vi "tacking_points.vi"(9 "NotifierReff":T1, 10 "Waypoint queue":refnum<queue>) -> (2 "size(s)":i32, 3 "New Sailing points":refnum<class "Waypoint.lvclass">[](array[class]), 5 "Waypoint Queue Out":refnum<queue>)   [LabVIEW 2013]
doc: "Creates tacking point or points nessisary to reach waypoint from current position. \n\n- (11/8/2014) Kaitlin Gallagher"
uses:
  Data/TypeDefs/Notifiers.ctl
  Data/TypeDefs/UTM Location.ctl
  Data/TypeDefs/Sail Set Suggestions.ctl
  Data/TypeDefs/Rudder Set Suggestions.ctl
  Data/TypeDefs/OverrideInformation.ctl
  Data/TypeDefs/OverrideMode.ctl
  Data/TypeDefs/MotorSetup.ctl
  Data/TypeDefs/DynamixelSetupInfo.ctl
  Data/TypeDefs/AirmarStatus.ctl
  Data/TypeDefs/HardwareOnline.ctl
  Data/TypeDefs/DynamixelCycleTracker.ctl
  Data/TypeDefs/RC Input Values.ctl
  Classes/Waypoint/Waypoint.lvclass
panel:
  in  "Coridor Width":dbl=100.0
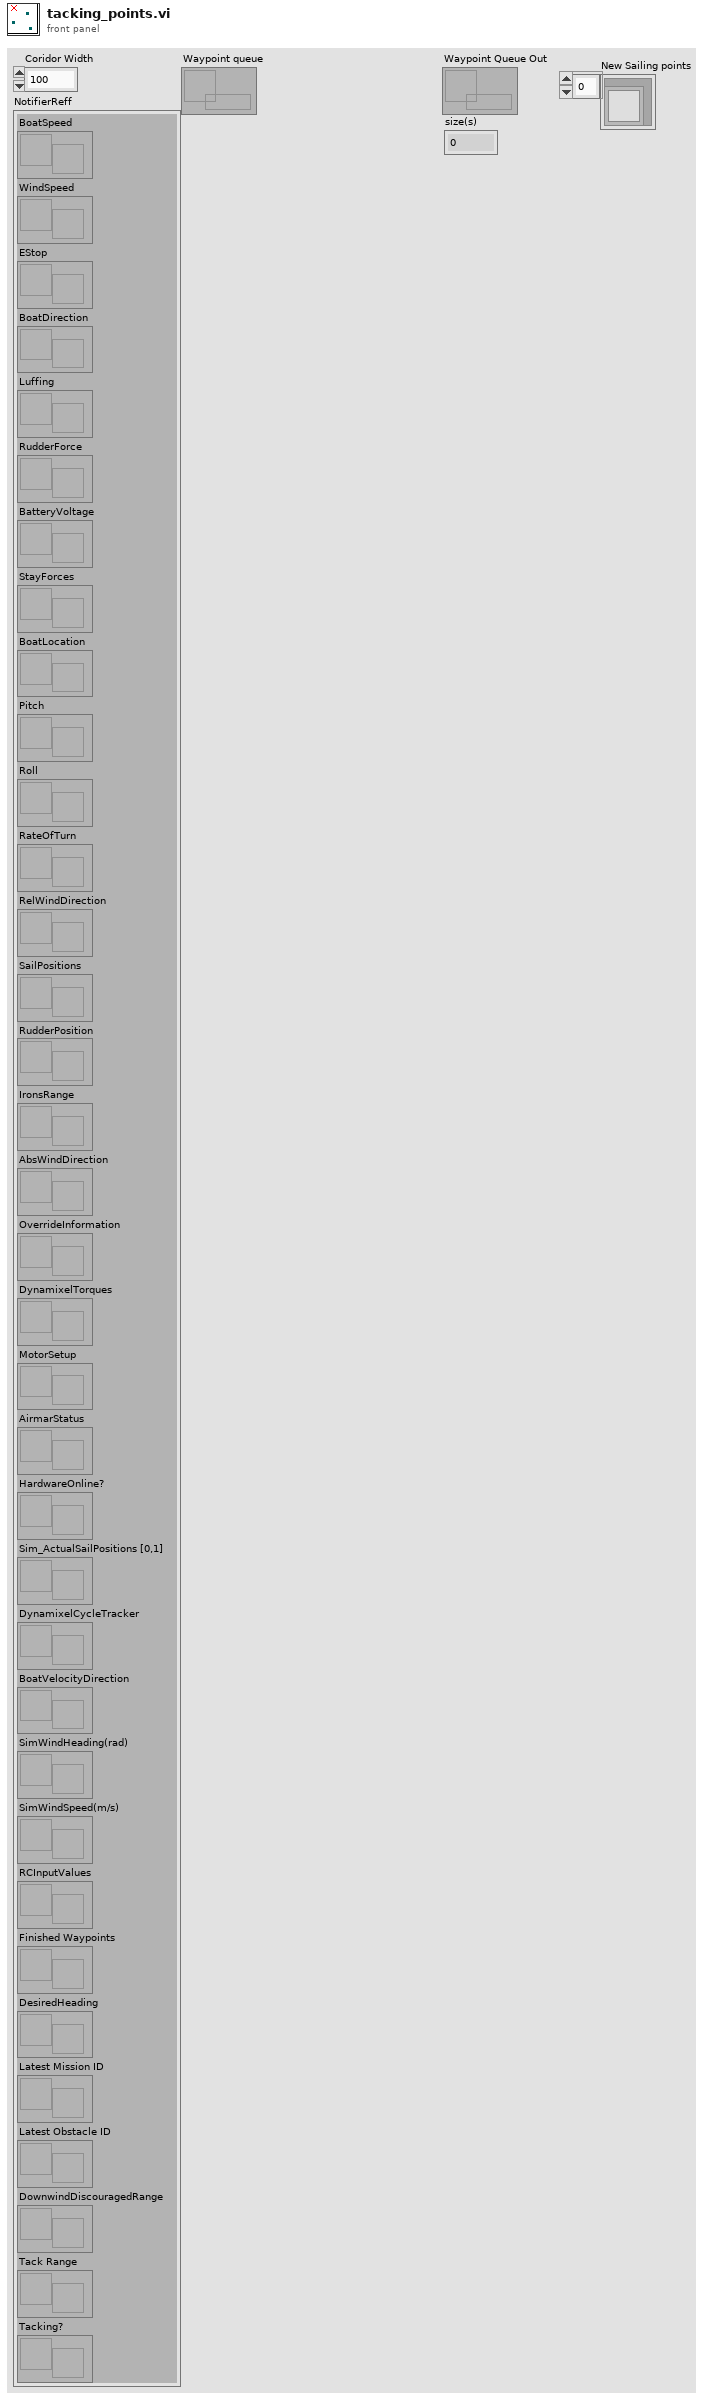
[diagram p1: front panel]
types:
  T1 = typedef "Notifiers.ctl" = cluster{"BoatSpeed":refnum<notifier>, "WindSpeed":refnum<notifier>, "EStop":refnum<notifier>, "BoatDirection":refnum<notifier>, "Luffing":refnum<notifier>, "RudderForce":refnum<notifier>, "BatteryVoltage":refnum<notifier>, "StayForces":refnum<notifier>, "BoatLocation":refnum<notifier>, "Pitch":refnum<notifier>, "Roll":refnum<notifier>, "RateOfTurn":refnum<notifier>, "RelWindDirection":refnum<notifier>, "SailPositions":refnum<notifier>, "RudderPosition":refnum<notifier>, "IronsRange":refnum<notifier>, "AbsWindDirection":refnum<notifier>, "OverrideInformation":refnum<notifier>, "DynamixelTorques":refnum<notifier>, "MotorSetup":refnum<notifier>, "AirmarStatus":refnum<notifier>, "HardwareOnline?":refnum<notifier>, "Sim_ActualSailPositions [0,1]":refnum<notifier>, "DynamixelCycleTracker":refnum<notifier>, "BoatVelocityDirection":refnum<notifier>, "SimWindHeading(rad)":refnum<notifier>, "SimWindSpeed(m/s)":refnum<notifier>, "RCInputValues":refnum<notifier>, "Finished Waypoints":refnum<notifier>, "DesiredHeading":refnum<notifier>, "Latest Mission ID":refnum<notifier>, "Latest Obstacle ID":refnum<notifier>, "DownwindDiscouragedRange":refnum<notifier>, "Tack Range":refnum<notifier>, "Tacking?":refnum<notifier>}
  T2 = typedef "UTM Location.ctl" = cluster{"UTM Zone":dbl, "Hemisphere":enum16{"North", "South"}, "East":dbl, "North":dbl}
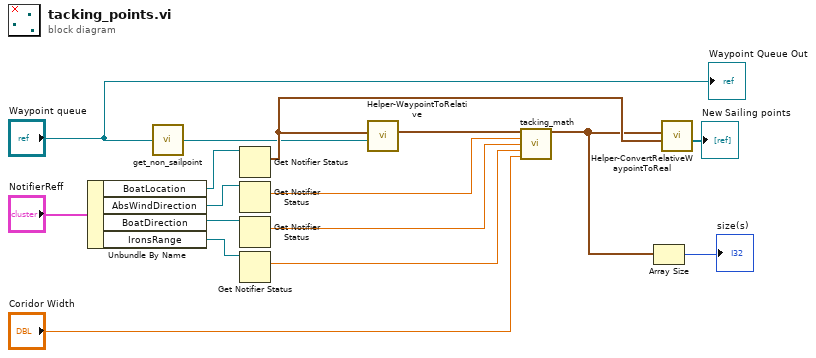
[diagram p0: block diagram]
diagram:
  n1 = Unbundle By Name("NotifierReff") -> ("BoatLocation"=w13:refnum<notifier>, "AbsWindDirection"=w12:refnum<notifier>, "BoatDirection"=w11:refnum<notifier>, "IronsRange"=w10:refnum<notifier>)
  n2 = call "get_non_sailpoint.vi"("Waypoint queue"="Waypoint queue") -> ("Waypoint Out"=w1:refnum<class "Waypoint.lvclass">)
  n3 = Get Notifier Status(notifier=w13) -> (current notification=w8:T2)  [unwired: 1 in, 4 out]
  n4 = Get Notifier Status(notifier=w12) -> (current notification=w3:dbl)  [unwired: 1 in, 4 out]
  n5 = Get Notifier Status(notifier=w11) -> (current notification=w4:dbl)  [unwired: 1 in, 4 out]
  n6 = Get Notifier Status(notifier=w10) -> (current notification=w9:dbl)  [unwired: 1 in, 4 out]
  n7 = call "Helper-WaypointToRelative.vi"("Next Waypoint"=w1, "Boat location"=w8) -> ("Relative Waypoint"=w16:cluster{"X":dbl, "Y":dbl})  [unwired: 9 in]
  n8 = call "tacking_math.vi"("Waypoint"=w16, "Wind Angle"=w3, "Boat Angle"=w4, "Irons Range"=w9, "Corridor Width"="Coridor Width") -> ("Sailling Pts"=w7:cluster{"X":dbl, "Y":dbl}[])  [unwired: 10 in]
  n9 = Array Size(array=w7) -> (size(s)=→"size(s)":i32)
  n10 = call "Helper-ConvertRelativeWaypointToReal.vi"("Current boat location"=w8, "Relative Waypoints In"=w7) -> ("Actual Waypoints Out"=→"New Sailing points":refnum<class "Waypoint.lvclass">[])  [unwired: 9 in]
  "Waypoint Queue Out" <- "Waypoint queue"
